vi "Read Child Attributes Map.vi"(11 "Core Actor in":refnum<class "Core Actor.lvclass">) -> (2 "Child Attributes Map":T1)   [LabVIEW 2025, in "jettl.lvlib" / "Core Actor.lvlib" / "Core Actor.lvclass"]
uses:
  Core Actor.lvclass
  Child Attributes Map.ctl
  Attributes/Attributes/Attributes.lvclass
  Core Actor.lvclass/Core Actor.ctl
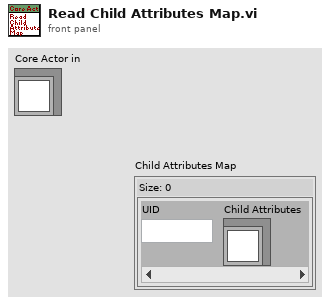
[diagram p1: front panel]
types:
  T1 = typedef "jettl.lvlib/Core Actor.lvlib/Core Actor.lvclass/Child Attributes Map.ctl" = map{string, refnum<class "Attributes.lvclass">}
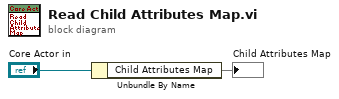
[diagram p0: block diagram]
diagram:
  n1 = Unbundle By Name("Core Actor in") -> ("Child Attributes Map"=→"Child Attributes Map":T1)
